vi "Agilent 3446X Series Acquire Single - Calibration.vi"(4 "Sim. Volt Set Point (V)":dbl format="%#_13g", 6 "Simulate":bool, 8 "error in (no error)":errorcluster, 9 "Absolute Resolution (1E-6)":dbl=1e-06, 10 "Measurement Function (10: Voltage DC)":i32(ring)=10 items=["Continuity", "Current AC", "Current DC", "Diode", "Frequency", "Resistance 4-wire", "Period", "Resistance 2-wire", "Temperature", "Voltage AC", "Voltage DC", "Voltage DC Ratio", "Capacitance"], 11 "VISA resource name":refnum<visa-resource-name>) -> (0 "error out":errorcluster, 3 "Measurement":dbl)   [LabVIEW 2023]
doc: "This example shows how to configure a measurement and take a reading."
uses:
  Agilent 3446X Series/Public/Data/Read (Single Point).vi
  Agilent 3446X Series/Agilent 3446X Series.lvlib
panel:
  in  "Manual Range (1)":dbl=1.0
  in  "Auto Range (T: Enable)":bool=TRUE
  # "(c) 2013-2021 National Instruments.  ALL RIGHTS RESERVED."
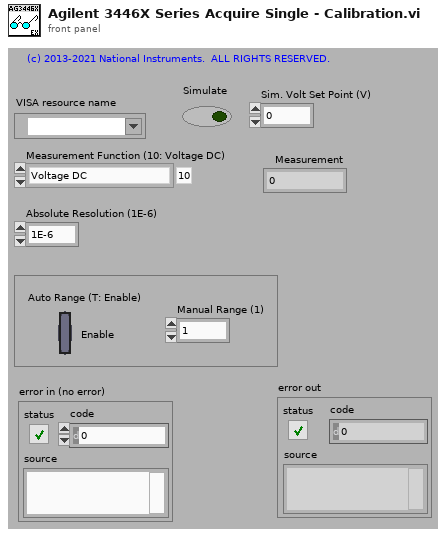
[diagram p1: front panel]
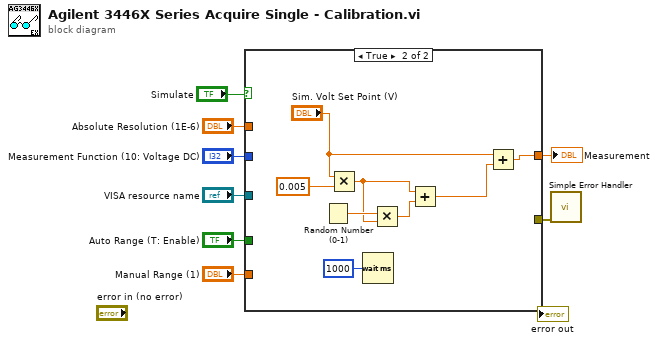
[diagram p0: block diagram]
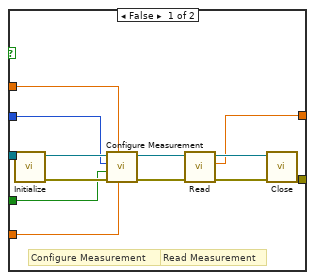
[diagram p2: hidden frame]
diagram:
  n1 = case shown="True" "Simulate" {
    tunnel: [w21 _] -> w8
    tunnel: [w14 w23] -> w7
    tunnel: "Auto Range (T: Enable)" -> [w13 _]
    tunnel: "Manual Range (1)" -> [w12 _]
    tunnel: "VISA resource name" -> [w11 _]
    tunnel: "Absolute Resolution (1E-6)" -> [w10 _]
    tunnel: "Measurement Function (10: Voltage DC)" -> [w9 _]
    frame False {
      # "Read Measurement"
      # "Configure Measurement"
      n2 = call "Initialize.vi"("VISA resource name"=w11) -> ("error out"=w19:errorcluster, "VISA resource name out"=w20:refnum<visa-resource-name>)  [unwired: 4 in, 5 out]
      n3 = call "Configure Measurement.vi"("Manual Range (1)"=w12, "Absolute Resolution (1E-6)"=w10, "error in (no error)"=w19, "Auto Range (T: Enable)"=w13, "Measurement Function (10: Voltage DC)"=w9, "VISA resource name"=w20) -> ("error out"=w15:errorcluster, "VISA resource name out"=w16:refnum<visa-resource-name>)  [unwired: 4 out]
      n4 = call-poly "Read.vi"("error in (no error)"=w15, "VISA resource name"=w16) -> ("error out"=w18:errorcluster, "Measurement"=w14:dbl, "VISA resource name out"=w17:refnum<visa-resource-name>)  [unwired: 7 out]
      n5 = call "Close.vi"("error in (no error)"=w18, "VISA resource name"=w17) -> ("error out"=w21:errorcluster)  [unwired: 9 out]
    }
    frame True {
      n6 = Random Number (0-1)() -> (number: 0 to 1=w28:dbl)
      n7 = Multiply(x="Sim. Volt Set Point (V)", y=0.005) -> (x*y=w24:dbl)
      n8 = Wait (ms)(milliseconds to wait=u32 1000) -> ()  [unwired: 1 out]
      n9 = Multiply(x=w28, y=w24) -> (x*y=w26:dbl)
      n10 = Add(x=w24, y=w26) -> (x+y=w25:dbl)
      n11 = Add(x="Sim. Volt Set Point (V)", y=w25) -> (x+y=w23:dbl)
    }
  }
  "Measurement" <- w7
  n12 = call <vilib>:"Simple Error Handler.vi"("error in (no error)"=w8) -> ()  [unwired: 1 in, 8 out]
